vi "Send.vi"(8 "error in (no error)":errorcluster, 10 "Message":refnum<class "BaseMessage.lvclass">, 11 "BaseReader in":refnum<class "BaseReader.lvclass">) -> (0 "error out":errorcluster, 2 "Sent Message":refnum<class "BaseMessage.lvclass">, 3 "BaseReader out":refnum<class "BaseReader.lvclass">)   [LabVIEW 2025, in "BaseReader.lvclass"]
doc: "Send a message to the remote destination"
uses:
  BaseReader.lvclass
  Message/BaseMessage/BaseMessage.lvclass
  BaseReader.lvclass/BaseReader.ctl
  Message/BaseMessage/BaseMessage.lvclass/BaseMessage.ctl
  Message/BaseMessage/Write Inherited timeout.vi
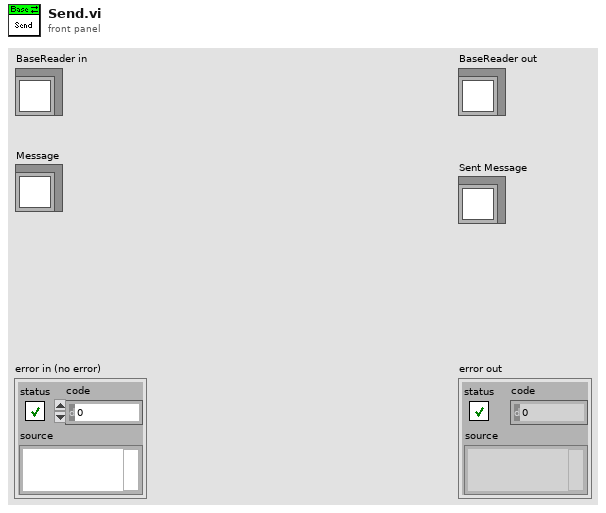
[diagram p1: front panel]
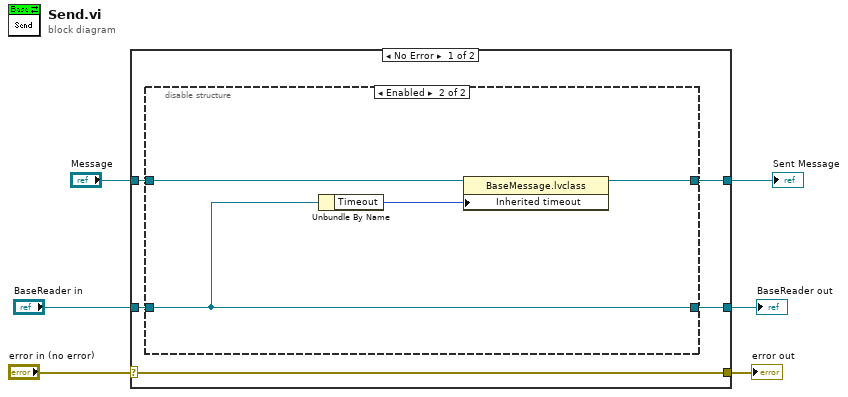
[diagram p0: block diagram]
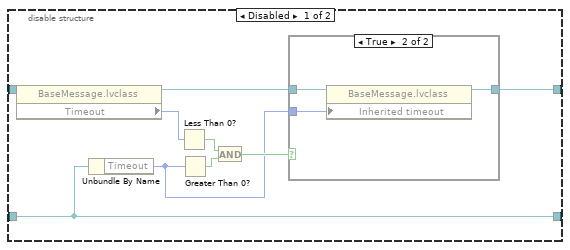
[diagram p2: hidden frame]
diagram:
  n1 = case shown="No Error" "error in (no error)" {
    selector: "error in (no error)" -> [w11 w31]
    tunnel: [w11 w31] -> w5
    tunnel: [w7 w30] -> w3
    tunnel: "BaseReader in" -> [w9 w30]
    tunnel: [w8 w29] -> w2
    tunnel: "Message" -> [w10 w29]
    frame No Error {
      n2 = disable-structure shown="Enabled" {
        disable-tunnel: w10 -> [w20 w26]
        disable-tunnel: w9 -> [w12 w25]
        disable-tunnel: [w15 w28] -> w8
        disable-tunnel: [w12 w25] -> w7
        frame Disabled {
          n3 = property on="Property Node" class="BaseMessage.lvclass"(reference=w20) -> (reference out=w19:refnum<class "BaseMessage.lvclass">, "Timeout"=w18:i32)  [unwired: 1 in, 1 out]
          n4 = Unbundle By Name(w12) -> ("Timeout"=w13:i32)
          n5 = Less Than 0?(x=w18) -> (x < 0?=w16:bool)
          n6 = Greater Than 0?(x=w13) -> (x > 0?=w17:bool)
          n7 = And(x=w16, y=w17) -> (x .and. y?=w14:bool)
          n8 = case shown="True" w14 {
            tunnel: w19 -> [w21 w24]
            tunnel: [w21 w23] -> w15
            tunnel: w13 -> [_ w22]
            frame False {
            }
            frame True {
              n9 = property on="Property Node" class="BaseMessage.lvclass"(reference=w24, "Inherited timeout"=w22) -> (reference out=w23:refnum<class "BaseMessage.lvclass">)  [unwired: 1 in, 1 out]
            }
          }
        }
        frame Enabled {
          n10 = Unbundle By Name(w25) -> ("Timeout"=w27:i32)
          n11 = property on="Property Node" class="BaseMessage.lvclass"(reference=w26, "Inherited timeout"=w27) -> (reference out=w28:refnum<class "BaseMessage.lvclass">)  [unwired: 1 in, 1 out]
        }
      }
    }
    frame Error {
    }
  }
  "error out" <- w5
  "BaseReader out" <- w3
  "Sent Message" <- w2
